vi "BusBase_New.vi"(7 "CreateMethod(CreateOrLookUpExisting)":T1(ring), 8 "ErrorIn":errorcluster, 10 "ObjectName":string, 11 "ReferenceIn":refnum<class "BusBase.lvclass">) -> (0 "ErrorOut":errorcluster, 1 "DVRRefOut":refnum<data-value>, 2 "NewObjectCreated":bool, 3 "ReferenceOut":refnum<class "BusBase.lvclass">)   [LabVIEW 2021, in "BusBase.lvlib" / "BusBase.lvclass"]
uses:
  BusBase.lvclass
  C:/Localdata/Projects/TriekselSoft/TriekselsoftApplicationFramework/Source/.Externals/Library_TAF_ApplicationFramework/TAFBaseGUI/TAFBaseGUI.lvclass
  protected/ObjectAttributes.ctl
  BusBase.lvclass/BusBase.ctl
  Library_TAF_ApplicationFramework/TAFBaseGUI/TAFBaseGUI.lvclass
  C:/Localdata/Projects/TriekselSoft/TriekselsoftApplicationFramework/Source/.Externals/Interface_UserInterface_IFrontPanel/IFrontPanel/IFrontPanel.lvclass
  C:/Localdata/Projects/TriekselSoft/TriekselsoftApplicationFramework/Source/IInterface/IInterface.lvclass
  C:/Localdata/Projects/TriekselSoft/TriekselsoftApplicationFramework/Source/.Externals/Interface_TAF_ITAFGUIActions/ITAFGUIActions/ITAFGUIActions.lvclass
  C:/Localdata/Projects/TriekselSoft/TriekselsoftApplicationFramework/Source/.Externals/Interface_Object_ICreateDestroy/ICreateDestroy/ICreateDestroy.lvclass
  C:/Localdata/Projects/TriekselSoft/TriekselsoftApplicationFramework/Source/.Externals/Interface_Object_IPersistentData/IPersistentData/IPersistentData.lvclass
  C:/Localdata/Projects/TriekselSoft/TriekselsoftApplicationFramework/Source/.Externals/Interface_TAF_ITAFObject/ITAFObject/ITAFObject.lvclass
  C:/Localdata/Projects/TriekselSoft/TriekselsoftApplicationFramework/Source/.Externals/Library_TAF_BusBase/BusBase/BusBase/BusBase.lvclass
panel:
  in  "DVRRef(Hidden)":refnum<data-value>
  in  "Data":T2
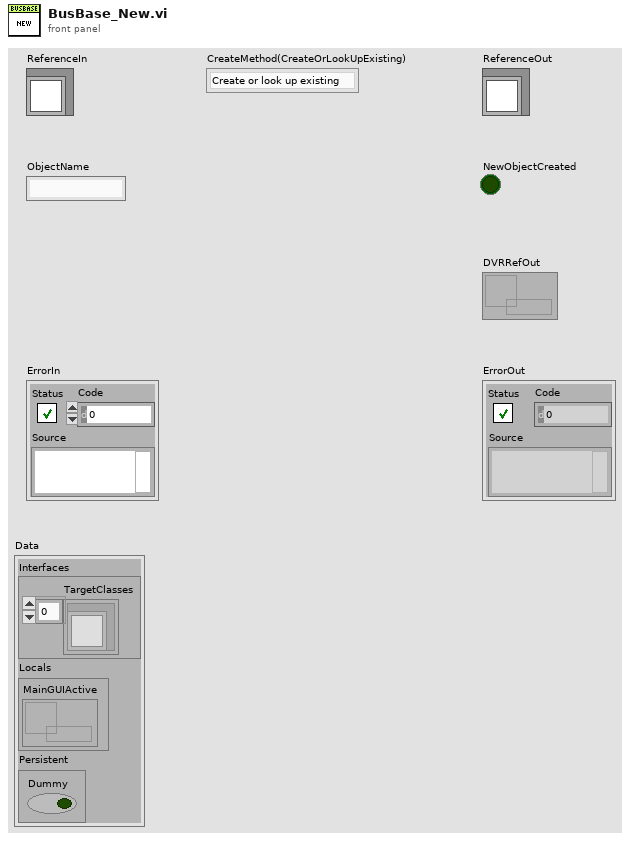
[diagram p1: front panel]
types:
  T1 = enum16{"Create or look up existing", "Look up existing"}
  T2 = typedef "BusBase.lvlib/BusBase.lvclass/ObjectAttributes.ctl" = cluster{"Interfaces":cluster{"TargetClasses":refnum<class>[]}, "Locals":cluster{"MainGUIActive":refnum<queue>}, "Persistent":cluster{"Dummy":bool}}
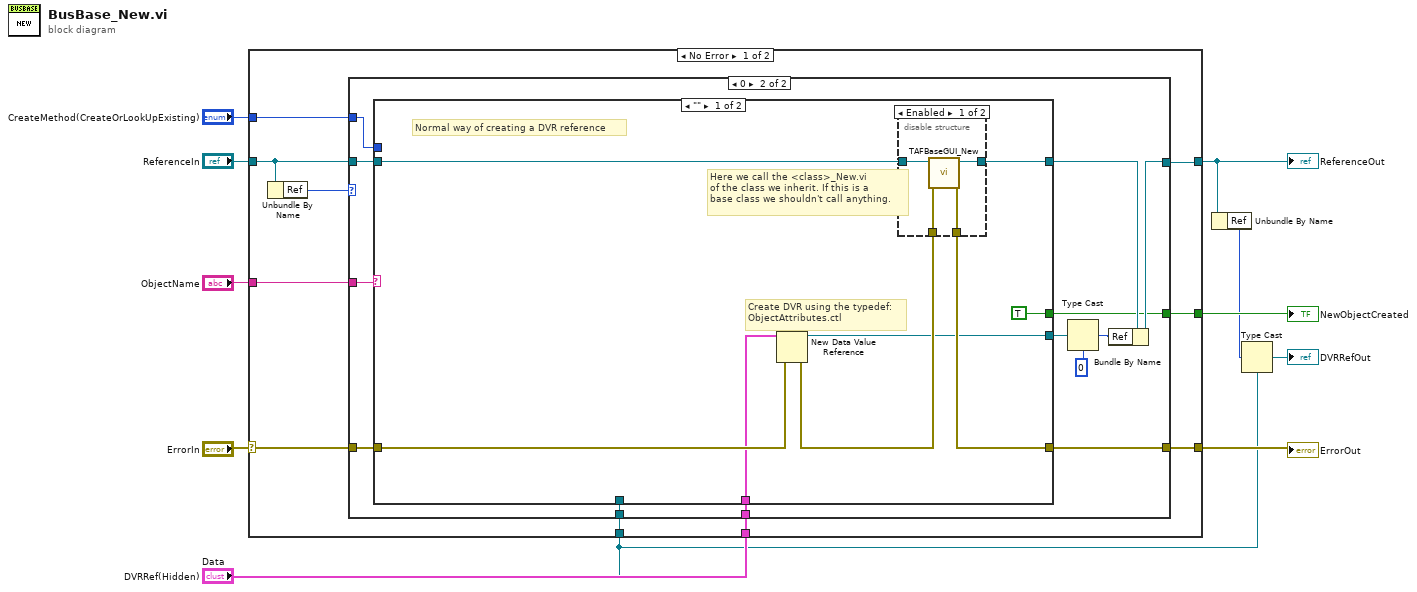
[diagram p0: block diagram]
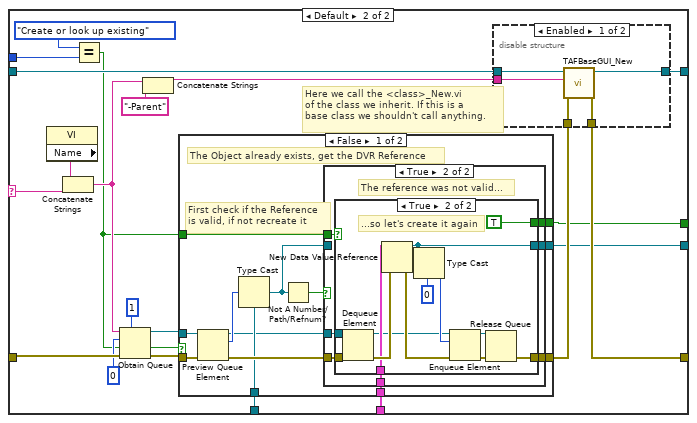
[diagram p4: hidden frame]
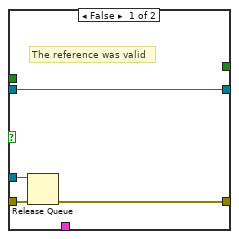
[diagram p5: hidden frame]
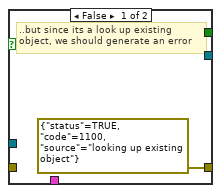
[diagram p6: hidden frame]
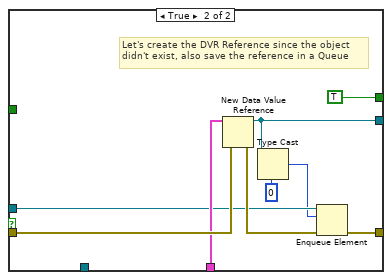
[diagram p7: hidden frame]
diagram:
  n1 = case shown="No Error" "ErrorIn" {
    selector: "ErrorIn" -> [w21 w128]
    tunnel: [w20 w128] -> w10
    tunnel: "CreateMethod(CreateOrLookUpExisting)" -> [w18 _]
    tunnel: "ObjectName" -> [w19 _]
    tunnel: "Data" -> [w17 _]
    tunnel: "DVRRef(Hidden)" -> [w16 _]
    tunnel: "ReferenceIn" -> [w15 w127]
    tunnel: [w14 w127] -> w4
    tunnel: [w13 _] -> w5
    frame No Error {
      n2 = Unbundle By Name(w15) -> ("Ref"=w12:u32)
      n3 = case shown="0" w12 {
        tunnel: w21 -> [w23 w36]
        tunnel: w19 -> [_ w34]
        tunnel: w18 -> [_ w33]
        tunnel: [w23 w35] -> w20
        tunnel: w17 -> [_ w32]
        tunnel: w15 -> [w22 w29]
        tunnel: [w22 w30] -> w14
        tunnel: w16 -> [_ w27]
        tunnel: [_ w26] -> w13
        frame Default {
          # "The DVR reference has already been created, from this child class's <Child>_New.vi"
        }
        frame 0 {
          n4 = case shown="\"\"" w34 {
            selector: w34 -> [_ w60]
            tunnel: w36 -> [w44 w71]
            tunnel: [w42 w72] -> w35
            tunnel: w33 -> [_ w67]
            tunnel: w32 -> [w41 w57]
            tunnel: [w40 w54] -> w31
            tunnel: w29 -> [w39 w66]
            tunnel: [w38 w65] -> w28
            tunnel: w27 -> [_ w58]
            tunnel: [TRUE w53] -> w26
            frame "" {
              # "Create DVR using the typedef:\nObjectAttributes.ctl"
              # "Here we call the <class>_New.vi\nof the class we inherit. If this is a\nbase class we shouldn't call anything."
              # "Normal way of creating a DVR reference"
              n5 = New Data Value Reference(data value=w41, error in=w44) -> (data value reference=w40:refnum<data-value>, error out=w43:errorcluster)
              n6 = disable-structure shown="Enabled" {
                disable-tunnel: w39 -> [w46 w49]
                disable-tunnel: [w45 w49] -> w38
                disable-tunnel: w43 -> [w48 w50]
                disable-tunnel: [w47 w50] -> w42
                frame Enabled {
                  n7 = call "TAFBaseGUI_New.vi"("ErrorIn"=w48, "ReferenceIn"=w46) -> ("ErrorOut"=w47:errorcluster, "ReferenceOut"=w45:refnum<class "BusBase.lvclass">)  [unwired: 6 in, 2 out]
                }
                frame Disabled {
                }
              }
            }
            frame Default {
              # "Here we call the <class>_New.vi\nof the class we inherit. If this is a\nbase class we shouldn't call anything."
              n8 = property class="VI"() -> ("Name"=w61:string)  [unwired: 2 in, 2 out]
              n9 = Concatenate Strings(w61, w60) -> (w59:string)
              n10 = Equal?(x=T1."Create or look up existing", y=w67) -> (x = y?=w52:bool)
              n11 = Obtain Queue(max queue size (-1, unlimited)=1, name (unnamed)=w59, element data type=u32 0 ("DataRef"), create if not found? (T)=w52, error in (no error)=w71) -> (queue out=w56:refnum<queue>, created new?=w55:bool, error out=w70:errorcluster)
              n12 = Concatenate Strings(w59, "-Parent" ("string")) -> (w62:string)
              n13 = case shown="False" w55 {
                tunnel: w70 -> [w85 w119]
                tunnel: w57 -> [w75 w116]
                tunnel: w56 -> [w82 w115]
                tunnel: [w83 w117] -> w69
                tunnel: [w77 w113] -> w54
                tunnel: w58 -> [w80 _]
                tunnel: [w74 TRUE] -> w53
                tunnel: w52 -> [w73 _]
                frame False {
                  # "First check if the Reference\nis valid, if not recreate it"
                  # "The Object already exists, get the DVR Reference"
                  n14 = Preview Queue Element(queue=w82, error in (no error)=w85) -> (queue out=w76:refnum<queue>, element=w81:u32, error out=w84:errorcluster)  [unwired: 1 in, 1 out]
                  n15 = Type Cast(type=w80, x=w81) -> (*(type *) &x=w78:refnum<data-value>)
                  n16 = Not A Number/Path/Refnum?(number/path/refnum=w78) -> (NaN/Path/Refnum?=w79:bool)
                  n17 = case shown="True" w79 {
                    tunnel: w84 -> [w89 w96]
                    tunnel: [w88 w95] -> w83
                    tunnel: w78 -> [w87 _]
                    tunnel: [w87 w92] -> w77
                    tunnel: w76 -> [w86 w94]
                    tunnel: w75 -> [_ w93]
                    tunnel: [_ w91] -> w74
                    tunnel: w73 -> [_ w90]
                    frame False {
                      # "The reference was valid"
                      n18 = Release Queue(queue=w86, error in (no error)=w89) -> (error out=w88:errorcluster)  [unwired: 1 in, 2 out]
                    }
                    frame True {
                      # "The reference was not valid..."
                      n19 = case shown="True" w90 {
                        tunnel: w94 -> [_ w105]
                        tunnel: w96 -> [_ w110]
                        tunnel: w93 -> [_ w102]
                        tunnel: [_ w100] -> w92
                        tunnel: [errorcluster {"status"=TRUE, "code"=1100, "source"="looking up existing object"} ("error out") w106] -> w95
                        tunnel: [_ TRUE] -> w91
                        frame False {
                          # "..but since its a look up existing\nobject, we should generate an error"
                        }
                        frame True {
                          # "...so let's create it again"
                          n20 = Dequeue Element(queue=w105, error in (no error)=w110) -> (queue out=w101:refnum<queue>, error out=w109:errorcluster)  [unwired: 1 in, 2 out]
                          n21 = New Data Value Reference(data value=w102, error in=w109) -> (data value reference=w100:refnum<data-value>, error out=w108:errorcluster)
                          n22 = Type Cast(type=u32 0 ("ObjectQueue"), x=w100) -> (*(type *) &x=w103:u32)
                          n23 = Enqueue Element(queue=w101, element=w103, error in (no error)=w108) -> (queue out=w98:refnum<queue>, error out=w107:errorcluster)  [unwired: 1 in, 1 out]
                          n24 = Release Queue(queue=w98, error in (no error)=w107) -> (error out=w106:errorcluster)  [unwired: 1 in, 2 out]
                        }
                      }
                    }
                  }
                }
                frame True {
                  # "Let's create the DVR Reference since the object\ndidn't exist, also save the reference in a Queue"
                  n25 = New Data Value Reference(data value=w116, error in=w119) -> (data value reference=w113:refnum<data-value>, error out=w118:errorcluster)
                  n26 = Type Cast(type=u32 0 ("ObjectQueue"), x=w113) -> (*(type *) &x=w112:u32)
                  n27 = Enqueue Element(queue=w115, element=w112, error in (no error)=w118) -> (error out=w117:errorcluster)  [unwired: 1 in, 2 out]
                }
              }
              n28 = disable-structure shown="Enabled" {
                disable-tunnel: w66 -> [w122 w125]
                disable-tunnel: [w121 w125] -> w65
                disable-tunnel: w62 -> [w120 _]
                disable-tunnel: w69 -> [w124 w126]
                disable-tunnel: [w123 w126] -> w72
                frame Enabled {
                  n29 = call "TAFBaseGUI_New.vi"("ErrorIn"=w124, "ObjectName"=w120, "ReferenceIn"=w122) -> ("ErrorOut"=w123:errorcluster, "ReferenceOut"=w121:refnum<class "BusBase.lvclass">)  [unwired: 5 in, 2 out]
                }
                frame Disabled {
                }
              }
            }
          }
          n30 = Type Cast(type=u32 0 ("DataRef"), x=w31) -> (*(type *) &x=w25:u32)
          n31 = Bundle By Name(cluster=w28, "Ref"=w25) -> (w30:refnum<class "BusBase.lvclass">)
        }
      }
    }
    frame Error {
    }
  }
  "ErrorOut" <- w10
  "ReferenceOut" <- w4
  "NewObjectCreated" <- w5
  n32 = Unbundle By Name(w4) -> ("Ref"=w3:u32)
  n33 = Type Cast(type="DVRRef(Hidden)", x=w3) -> (*(type *) &x=→"DVRRefOut":refnum<data-value>)
